vi "wasSuccessful.vi"(8 "error in (no error)":errorcluster, 11 "TestResult in":refnum<class "TestResult.lvclass">) -> (0 "error out":errorcluster, 2 "successful?":bool, 3 "TestResult in":refnum<class "TestResult.lvclass">)   [LabVIEW 2013, in "TestResult.lvclass"]
uses:
  TestResult.lvclass
  TestResult.lvclass/TestResult.ctl
panel:
  # "JKI VI Tester for LabVIEW\nhttp://jkisoft.com/vi-tester\nCopyright (C) 2007-2009, JKI <info@jkisoft.com>\nALL RIGHTS RESERVED"
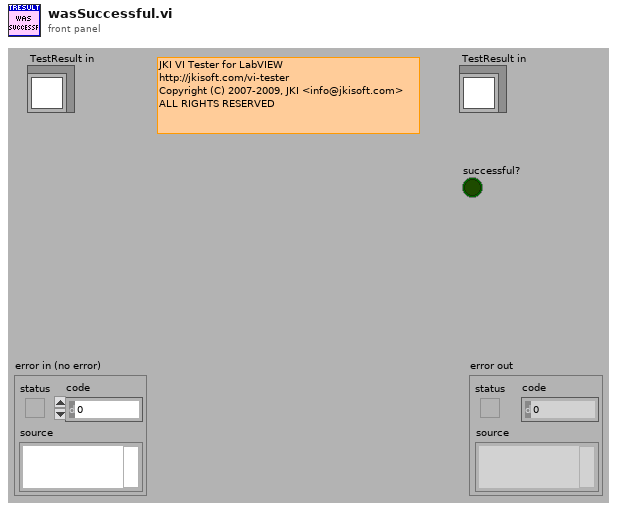
[diagram p1: front panel]
types:
  T1 = typedef "TestResult.lvclass/errors.ctl" = T2[]
  T2 = typedef "TestResult.lvclass/error.ctl" = cluster{"test":refnum<class>, "error":errorcluster}
  T3 = typedef "TestResult.lvclass/failure.ctl" = cluster{"test":refnum<class>, "error":errorcluster}
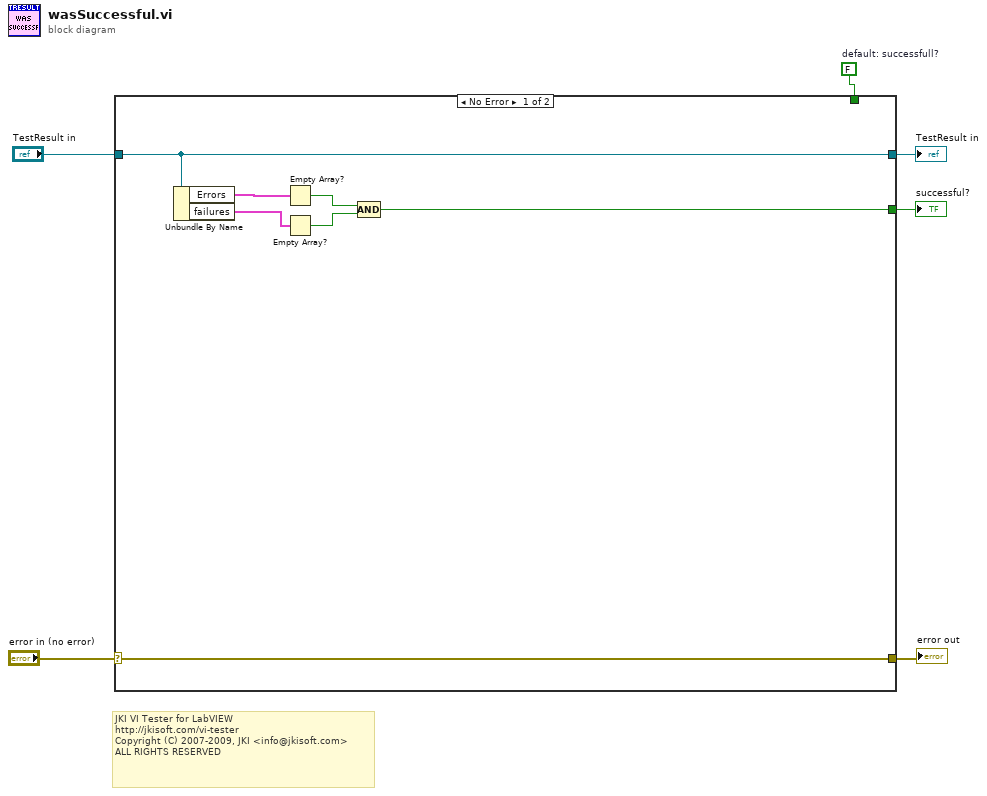
[diagram p0: block diagram]
diagram:
  w1 = FALSE  # default: successfull?
  # "JKI VI Tester for LabVIEW\nhttp://jkisoft.com/vi-tester\nCopyright (C) 2007-2009, JKI <info@jkisoft.com>\nALL RIGHTS RESERVED"
  n1 = case shown="No Error" "error in (no error)" {
    selector: "error in (no error)" -> [w13 w16]
    tunnel: [w13 w16] -> w5
    tunnel: [w12 w15] -> w3
    tunnel: "TestResult in" -> [w12 w15]
    tunnel: [w7 w14] -> w2
    tunnel: w1 -> [_ w14]
    frame No Error {
      n2 = Unbundle By Name(w12) -> ("Errors"=w11:T1, "failures"=w10:T3[])
      n3 = Empty Array?(array=w11) -> (empty?=w9:bool)
      n4 = Empty Array?(array=w10) -> (empty?=w8:bool)
      n5 = Compound Arithmetic op=AND(w9, w8) -> (w7:bool)
    }
    frame Error {
    }
  }
  "error out" <- w5
  "TestResult in" <- w3
  "successful?" <- w2
